vi "FeedbackDecode_Params2Preset.vi"(2 "StimClustIn":T1={"ParamsTable"=[], "Sel"=[], "Stim"=FALSE, "StimMode"=enum."Off", "StimStep"=[enum."1uA", enum."1uA", enum."Off"], "Jitter"=FALSE, "Pulse"=FALSE, "BFreq"=0.0, "BAmp"=0.0, "UEAArray"=[], "AdjClust"={"Add"=FALSE, "Sub"=FALSE, "Val"=[1.0, 100.0, 0.2, 500.0, 0.0], "B"=[FALSE, FALSE, FALSE, FALSE, FALSE], "Inc+"=["x+1", "x+10", "x+0.1", "x+10", "x+10"], "Set"=FALSE, "LoadTable"=FALSE, "SaveTable"=FALSE, "ClearTable"=FALSE, "DeleteSel"=FALSE, "Inc-"=["x-1", "x-10", "x-0.1", "x-10", "x-10"]}, "PresetTable"=[], "SelPreset"=[], "SortClust"={"Region"=FALSE, "Receptor"=FALSE, "Electrode"=FALSE, "Min Amp"=FALSE, "Max Amp"=FALSE, "Min Freq"=FALSE, "Max Freq"=FALSE, "Duration"=FALSE}, "SelSort"={"Sel"=FALSE}, "PresetClust"={"Load"=FALSE, "Clear"=FALSE, "Save"=FALSE, "Del"=FALSE}, "RespClust"={"RespType"=enum."Sensor Map", "OpenResp"=FALSE}, "AmpLimit"=0.0, "FreqLimit"=0.0, "DurLimit"=0.0, "Wait Period"=0.0, "Train Period"=0.0} {"Train Period" min=0.0 max=100.0 step=0.1; "Wait Period" min=0.0 max=100.0 step=0.1; "DurLimit" min=0.0 max=1.0 step=0.01; "FreqLimit" min=0.0 max=500.0 step=1.0; "AmpLimit" min=0.0 max=100.0 step=1.0; "BAmp" min=0.0 max=100.0 step=1.0; "BFreq" min=0.0 max=100.0 step=1.0}) -> (0 "StimClustOut":T1={"ParamsTable"=[], "Sel"=[], "Stim"=FALSE, "StimMode"=enum."Off", "StimStep"=[enum."1uA", enum."1uA", enum."Off"], "Jitter"=FALSE, "Pulse"=FALSE, "BFreq"=0.0, "BAmp"=0.0, "UEAArray"=[], "AdjClust"={"Add"=FALSE, "Sub"=FALSE, "Val"=[1.0, 100.0, 0.2, 500.0, 0.0], "B"=[FALSE, FALSE, FALSE, FALSE, FALSE], "Inc+"=["x+1", "x+10", "x+0.1", "x+10", "x+10"], "Set"=FALSE, "LoadTable"=FALSE, "SaveTable"=FALSE, "ClearTable"=FALSE, "DeleteSel"=FALSE, "Inc-"=["x-1", "x-10", "x-0.1", "x-10", "x-10"]}, "PresetTable"=[], "SelPreset"=[], "SortClust"={"Region"=FALSE, "Receptor"=FALSE, "Electrode"=FALSE, "Min Amp"=FALSE, "Max Amp"=FALSE, "Min Freq"=FALSE, "Max Freq"=FALSE, "Duration"=FALSE}, "SelSort"={"Sel"=FALSE}, "PresetClust"={"Load"=FALSE, "Clear"=FALSE, "Save"=FALSE, "Del"=FALSE}, "RespClust"={"RespType"=enum."Sensor Map", "OpenResp"=FALSE}, "AmpLimit"=0.0, "FreqLimit"=0.0, "DurLimit"=0.0, "Wait Period"=0.0, "Train Period"=0.0} {"Train Period" min=0.0 max=100.0 step=0.1; "Wait Period" min=0.0 max=100.0 step=0.1; "DurLimit" min=0.0 max=1.0 step=0.01; "FreqLimit" min=0.0 max=500.0 step=1.0; "AmpLimit" min=0.0 max=100.0 step=1.0; "BAmp" min=0.0 max=100.0 step=1.0; "BFreq" min=0.0 max=100.0 step=1.0})   [LabVIEW 2020]
uses:
  FeedbackDecode_EncodeClust.ctl
  <vilib>/regexp/Match Regular Expression.xnode
panel:
  # "Value"
  # "Inc-"
  # "Inc+"
  # "Min Amp"
  # "Max Amp"
  # "Min Freq"
  # "Max Freq"
  # "Duration"
  # "Value"
  # "Inc-"
  # "Inc+"
  # "Min Amp"
  # "Max Amp"
  # "Min Freq"
  # "Max Freq"
  # "Duration"
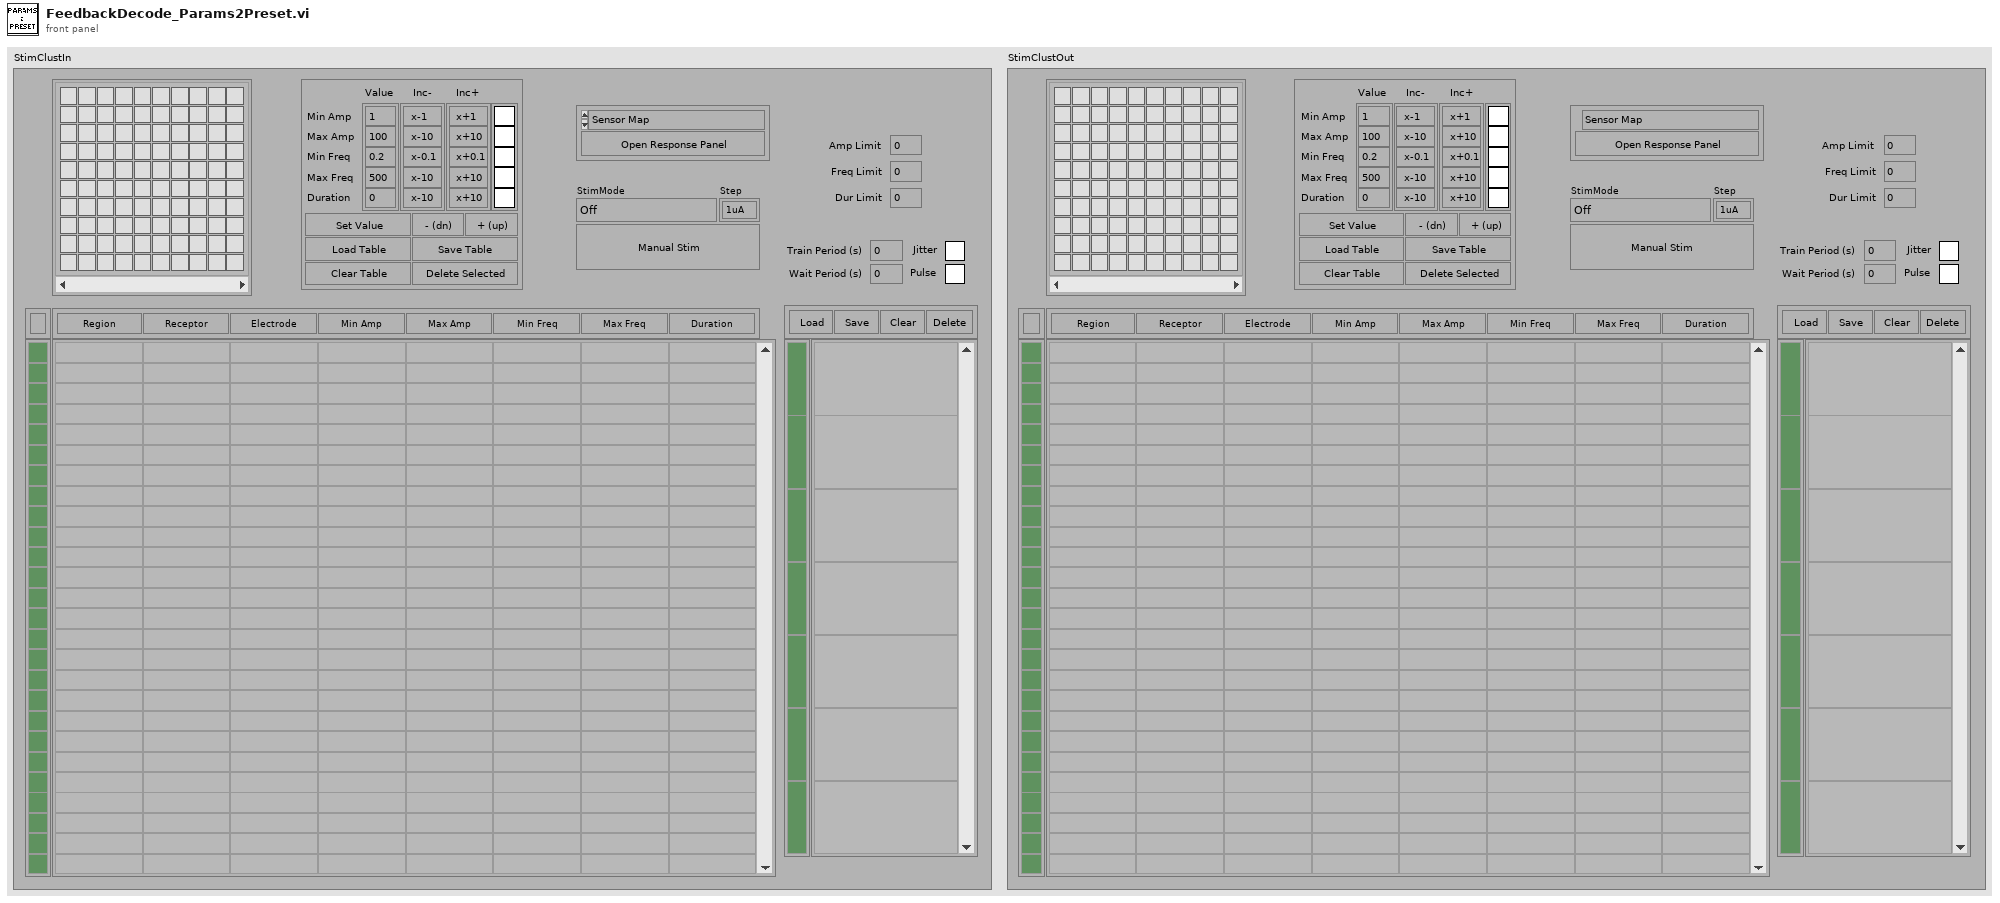
[diagram p1: front panel]
types:
  T1 = typedef "FeedbackDecode_EncodeClust.ctl" = cluster{"ParamsTable":string[][], "Sel":bool[], "Stim":bool, "StimMode":enum16{"Off", "Manual", "MSMS", "VRE", "3DHand", "DEKA", "Analog(DEKA)"}, "StimStep":enum16{"Off", "1uA", "2uA", "5uA", "10uA", "20uA", "30uA"}[], "Jitter":bool, "Pulse":bool, "BFreq":dbl, "BAmp":dbl, "UEAArray":cluster{"Boolean 1":bool, "Boolean 2":bool, "Boolean 3":bool, "Boolean 4":bool, "Boolean 5":bool, "Boolean 6":bool, "Boolean 7":bool, "Boolean 8":bool, "Boolean 9":bool, "Boolean 10":bool, "Boolean 11":bool, "Boolean 12":bool, "Boolean 13":bool, "Boolean 14":bool, "Boolean 15":bool, "Boolean 16":bool, "Boolean 17":bool, "Boolean 18":bool, "Boolean 19":bool, "Boolean 20":bool, "Boolean 21":bool, "Boolean 22":bool, "Boolean 23":bool, "Boolean 24":bool, "Boolean 25":bool, "Boolean 26":bool, "Boolean 27":bool, "Boolean 28":bool, "Boolean 29":bool, "Boolean 30":bool, "Boolean 31":bool, "Boolean 32":bool, "Boolean 33":bool, "Boolean 34":bool, "Boolean 35":bool, "Boolean 36":bool, "Boolean 37":bool, "Boolean 38":bool, "Boolean 39":bool, "Boolean 40":bool, "Boolean 41":bool, "Boolean 42":bool, "Boolean 43":bool, "Boolean 44":bool, "Boolean 45":bool, "Boolean 46":bool, "Boolean 47":bool, "Boolean 48":bool, "Boolean 49":bool, "Boolean 50":bool, "Boolean 51":bool, "Boolean 52":bool, "Boolean 53":bool, "Boolean 54":bool, "Boolean 55":bool, "Boolean 56":bool, "Boolean 57":bool, "Boolean 58":bool, "Boolean 59":bool, "Boolean 60":bool, "Boolean 61":bool, "Boolean 62":bool, "Boolean 63":bool, "Boolean 64":bool, "Boolean 65":bool, "Boolean 66":bool, "Boolean 67":bool, "Boolean 68":bool, "Boolean 69":bool, "Boolean 70":bool, "Boolean 71":bool, "Boolean 72":bool, "Boolean 73":bool, "Boolean 74":bool, "Boolean 75":bool, "Boolean 76":bool, "Boolean 77":bool, "Boolean 78":bool, "Boolean 79":bool, "Boolean 80":bool, "Boolean 81":bool, "Boolean 82":bool, "Boolean 83":bool, "Boolean 84":bool, "Boolean 85":bool, "Boolean 86":bool, "Boolean 87":bool, "Boolean 88":bool, "Boolean 89":bool, "Boolean 90":bool, "Boolean 91":bool, "Boolean 92":bool, "Boolean 93":bool, "Boolean 94":bool, "Boolean 95":bool, "Boolean 96":bool, "Boolean 97":bool, "Boolean 98":bool, "Boolean 99":bool, "Boolean 100":bool}[], "AdjClust":cluster{"Add":bool, "Sub":bool, "Val":dbl[], "B":bool[], "Inc+":string[], "Set":bool, "LoadTable":bool, "SaveTable":bool, "ClearTable":bool, "DeleteSel":bool, "Inc-":string[]}, "PresetTable":string[][], "SelPreset":bool[], "SortClust":cluster{"Region":bool, "Receptor":bool, "Electrode":bool, "Min Amp":bool, "Max Amp":bool, "Min Freq":bool, "Max Freq":bool, "Duration":bool}, "SelSort":cluster{"Sel":bool}, "PresetClust":cluster{"Load":bool, "Clear":bool, "Save":bool, "Del":bool}, "RespClust":cluster{"RespType":enum16{"Sensor Map", "Full Map"}, "OpenResp":bool}, "AmpLimit":dbl, "FreqLimit":dbl, "DurLimit":dbl, "Wait Period":dbl, "Train Period":dbl}
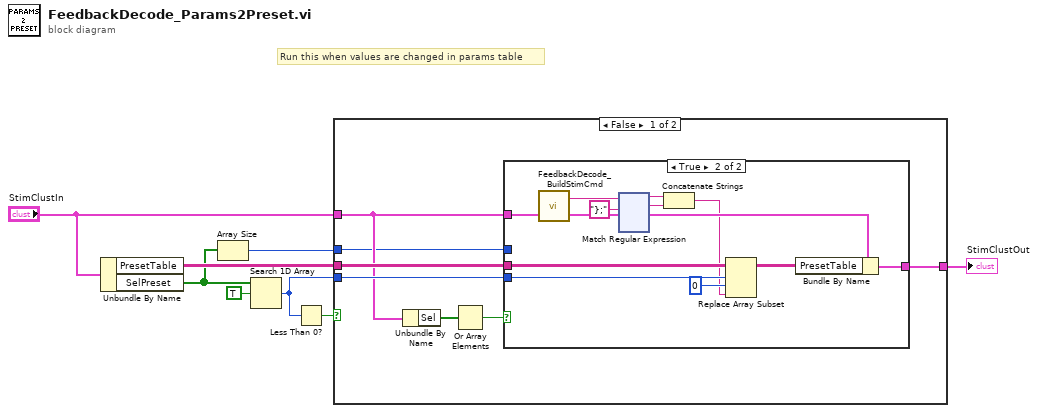
[diagram p0: block diagram]
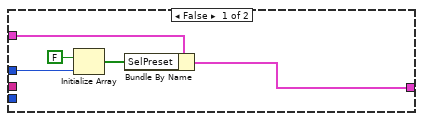
[diagram p2: hidden frame]
diagram:
  # "Run this when values are changed in params table"
  n1 = Unbundle By Name("StimClustIn") -> ("PresetTable"=w6:string[][], "SelPreset"=w2:bool[])
  n2 = Array Size(array=w2) -> (size(s)=w1:i32)
  n3 = Search 1D Array(1D array=w2, element=TRUE) -> (index of element=w3:i32)  [unwired: 1 in]
  n4 = Less Than 0?(x=w3) -> (x < 0?=w4:bool)
  n5 = case shown="False" w4 {
    tunnel: [w15 w147] -> w7
    tunnel: w6 -> [w14 _]
    tunnel: w3 -> [w13 _]
    tunnel: "StimClustIn" -> [w12 w147]
    tunnel: w1 -> [w9 _]
    frame False {
      n6 = Unbundle By Name(w12) -> ("Sel"=w11:bool[])
      n7 = Or Array Elements(Boolean array=w11) -> (logical OR=w10:bool)
      n8 = case shown="True" w10 {
        tunnel: [w16 w32] -> w15
        tunnel: w14 -> [_ w31]
        tunnel: w13 -> [_ w30]
        tunnel: w12 -> [w20 w26]
        tunnel: w9 -> [w19 _]
        frame False {
          n9 = Initialize Array(FALSE, w19) -> (w18:bool[])
          n10 = Bundle By Name(cluster=w20, "SelPreset"=w18) -> (w16:T1)
        }
        frame True {
          n11 = call "FeedbackDecode_BuildStimCmd.vi"("EncodeClustIn"=w26) -> ("EncodeClustOut"=w29:T1, "StimCmd"=w22:string)  [unwired: 1 in]
          n12 = xnode "Match Regular Expression"("input string"=w22, "regular expression"="};") -> ("before match"=w24:string, "whole match"=w25:string)  [unwired: 4 in, 3 out]
          n13 = Concatenate Strings(w24, w25) -> (w21:string)
          n14 = Replace Array Subset(array=w31, new element=w21, index (row)=w30, index (col)=0 ("disabled index (col)")) -> (w27:string[][])
          n15 = Bundle By Name(cluster=w29, "PresetTable"=w27) -> (w32:T1)
        }
      }
    }
    frame True {
    }
  }
  "StimClustOut" <- w7
